vi "Fluke 5XXX Series Multicalibrators Temperature Measurement.vi"() -> ()   [LabVIEW 2014]
doc: "The VI shows as example how to take one temperature measurement at a time. Following VIs are called:\n\n(1) Reset (reset):\nThis VI resets the instrument to a known state.\n\n(2) Set TC Type (setTCType):\nThis VI sets the Thermocouple (TC) temperature sensor type.\n\n(3) Set Thermocouple Meas Mode (setThermocoupleMeasMode):\nThis VI selects mode to measure the thermocouple temperature that is attached to the Calibrator TC terminals.\n\n(4) Wait-to-Continue (waitToContinue):\nThis VI Prevents further remote commands from being executed until all previous remote commands have been executed.\n\n(5) Get Thermocouple Meas Value (getThermocoupleMeasValue):\nThis VI returns the last value of the thermocouple measurement.\n\nRange checking, instrument model checking and option checking is performed by each of used VIs internaly. To skip instrument model checking, option checking and error checking, call VI\n\n FL5XMCAL State Checking.vi\n\nand disable it. When state checking is disabled driver does not check for correct instrument model or option to be used with each of VIs. This might cause unexpected behaviour of the instrument. Simpliest way how to disable state checking from the begining is calling initialization VI with the parameter ID Query = FALSE. But this is not recommended as functionality of the driver depends on the instrument models and its options.\n\nNotes:\n\n(1) Refer also to the descriptions of used VIs.\n\n(2) This VI is available only for instrument models 5500A and 5520A."
uses:
  Fluke 5XXX Series Multicalibrators.lvlib
panel:
  in  "Temperature Units (22: Temperature in degrees Celsius)":u32(ring)=22 items=["Unitless", "Frequency in units of hertz", "Frequency in units of kilohertz", "Frequency in units of megahertz", "Volts in units of microvolts", "Volts in units of millivolts", "Volts in units of volts", "Volts in units of kilovolts", "Current in units of microamperes", "Current in units of milliamps", "Current in units of amps", "Percent", "Parts-per-million", "Volts in units of decibels referenced to 1 milliwatt into 600 W load", "Resistance in units of ohms", "Resistance in units of kilohms", "Resistance in units of megohms", "Capacitance in units of nanofarads", "Capacitance in units of picofarads", "Capacitance in units of  microfarads", "Capacitance in units of millifarads", "Capacitance in units of farads", "Temperature in degrees Celsius", "Temperature in degrees Fahrenheit", "Period in units of nanoseconds", "Period in units of microseconds", "Period in units of milliseconds", "Period in units of seconds", "Pound-force pre square inch", "Meters of mercury", "Inches of mercury", "Inches of water", "Feet of water", "Meters of water", "Bar", "Pascal", "Grams per centimeter squared", "Inches of water @ 60 degrees Farhenheit", "Decibels"]
  in  "VISA resource name":refnum<visa-resource-name>
  out "Value Units":i32
  out "Meas Value":dbl format="%^.3e"
  in  "Thermocouple Type (4: K)":u32(ring)=4 items=["B", "C", "E", "J", "K", "L:Jdin", "N", "R", "S", "T", "U:Tdin", "X", "Y", "Z"]
  # "(c) 2005-2012 National Instruments.  ALL RIGHTS RESERVED."
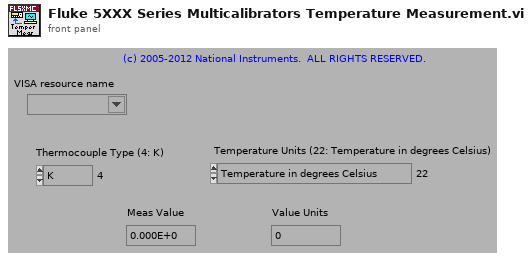
[diagram p1: front panel]
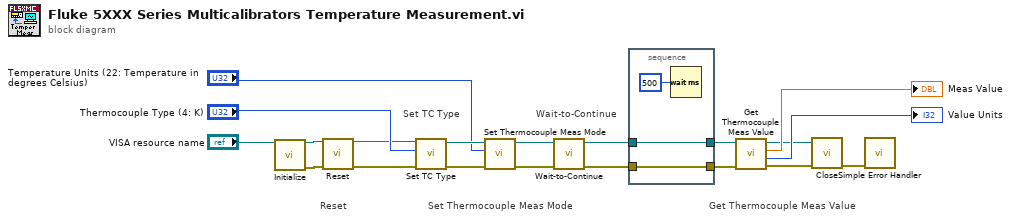
[diagram p0: block diagram]
diagram:
  # "Get Thermocouple Meas Value"
  # "Wait-to-Continue"
  # "Set Thermocouple Meas Mode"
  # "Set TC Type"
  # "Reset"
  n1 = call "Initialize.vi"("VISA resource name"="VISA resource name") -> ("VISA resource name out"=w2:refnum<visa-resource-name>, "error out"=w1:errorcluster)  [unwired: 13 in]
  n2 = call "Reset.vi"("VISA resource name"=w2, "error in (no error)"=w1) -> ("VISA resource name out"=w15:refnum<visa-resource-name>, "error out"=w20:errorcluster)  [unwired: 12 in]
  n3 = call "Set TC Type.vi"("error in (no error)"=w20, "Thermocouple Type (4: K)"="Thermocouple Type (4: K)", "VISA resource name"=w15) -> ("error out"=w19:errorcluster, "VISA resource name out"=w14:refnum<visa-resource-name>)  [unwired: 7 in]
  n4 = call "Set Thermocouple Meas Mode.vi"("error in (no error)"=w19, "Temperature Units (22: Temperature in degrees Celsius)"="Temperature Units (22: Temperature in degrees Celsius)", "VISA resource name"=w14) -> ("error out"=w18:errorcluster, "VISA resource name out"=w13:refnum<visa-resource-name>)  [unwired: 7 in]
  n5 = call "Wait-to-Continue.vi"("error in (no error)"=w18, "VISA resource name"=w13) -> ("error out"=w12:errorcluster, "VISA resource name out"=w10:refnum<visa-resource-name>)  [unwired: 8 in]
  n6 = stacked-sequence {
    tunnel: [w23] -> w11
    tunnel: w12 -> [w23]
    tunnel: [w22] -> w9
    tunnel: w10 -> [w22]
    frame #0 {
      n7 = Wait (ms)(milliseconds to wait=u32 500) -> ()  [unwired: 1 out]
    }
  }
  n8 = call "Get Thermocouple Meas Value.vi"("error in (no error)"=w11, "VISA resource name"=w9) -> ("error out"=w5:errorcluster, "Value Units"=→"Value Units":i32, "Meas Value"=→"Meas Value":dbl, "VISA resource name out"=w4:refnum<visa-resource-name>)  [unwired: 6 in]
  n9 = call "Close.vi"("VISA resource name"=w4, "error in (no error)"=w5) -> ("error out"=w6:errorcluster)  [unwired: 13 in]
  n10 = call <vilib>:"Simple Error Handler.vi"("error in (no error)"=w6) -> ()  [unwired: 4 in, 5 out]
